vi "Ymodem Constant.vi"(4 "Constant Defined":u8(ring)=1 items=["SOH"=1, "STX"=2, "ETX"=3, "EOF"=4, "ENQ"=5, "ACK"=6, "NAK"=21, "CAN"=24, "C"=67]) -> ()   [LabVIEW 2013]
doc: "Define the constant of the Ymodem protocol."
panel:
  # "SOH = 0x01 数据包开始\nSTX = 0x02 正文开始\nETX = 0x03 正文结束\nEOF= 0x04 数据包结束\nENQ = 0x05 询问字符\nACK = 0x06 确认\nNAK = 0x15 无应答 \nCAN = 0x18 取消传输\nC =0x43 进入开始传输状态"
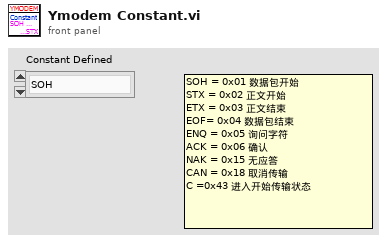
[diagram p1: front panel]
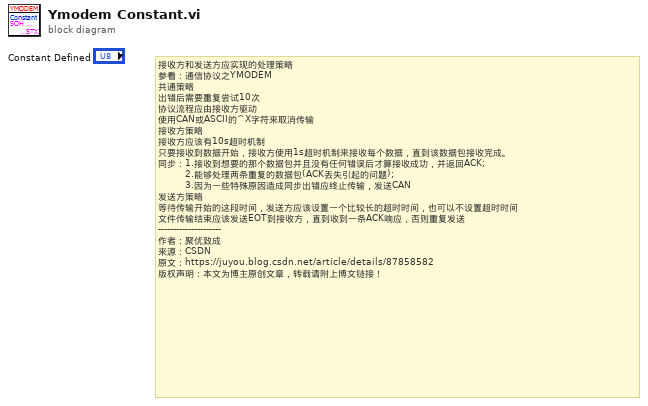
[diagram p0: block diagram]
diagram:
  # "接收方和发送方应实现的处理策略\n参看：通信协议之YMODEM\n共通策略\n出错后需要重复尝试10次\n协议流程应由接收方驱动\n使用CAN或ASCII的^X字符来取消传输\n接收方策略\n接收方应该有10s超时机制\n只要接收到数据开始，接收方使用1s超时机制来接收每个数据，直到该数据包接收完成。\n同步：1.接收到想要的那个数据包并且没有任何错误后才算接收成功，并返回ACK; \n         2.能够处理两条重复的数据包(ACK丢失引起的问题); \n         3.因为一些特殊原因造成同步出错应终止传输，发送CAN\n发送方策略\n等待传输开始的这段时间，发送方应该设置一个比较长的超时时间，也可以不设置超时时间\n文件传输结束应该发送EOT到接收方，直到收到一条ACK响应，否则重复发送\n--------------------- \n作者：聚优致成 \n来源：CSDN \n原文：https://juyou.blog.csdn.net/article/details/87858582 \n版权声明：本文为博主原创文章，转载请附上博文链接！"
